vi "LVRun 6.1.vi"() -> ()   [LabVIEW 2012]
panel:
  in  "quit? (T)\nCase Constant\n(See Context Help)":bool=TRUE
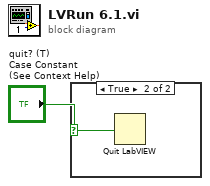
[diagram p0: block diagram]
diagram:
  n1 = case shown="True" "quit? (T)\nCase Constant\n(See Context Help)" {
    selector: "quit? (T)\nCase Constant\n(See Context Help)" -> [_ w2]
    frame False {
    }
    frame True {
      n2 = Quit LabVIEW(quit? (T)=w2) -> ()
    }
  }
